vi "sv_UFF58 Set Ordinate Unit and Label.vi"(0 "engineering units":T1=1 items=["custom..."=0, "V"=1, "A"=21, "C"=30, "pC"=31, "s"=32, "-"=29, "Pa"=2, "N"=20, "g"=3, "m/s^2"=4, "m/s"=5, "m"=6, "mm/s"=12, "mm"=13, "micron/s"=14, "micron"=15, "in/s^2"=7, "in/s"=8, "in"=9, "mil/s"=10, "mil"=11, "rad/s^2"=16, "rad/s"=17, "rad"=18, "deg/s^2"=26, "deg/s"=27, "deg"=28, "RPM"=22, "cycle/s^2"=23, "Hz"=24, "cycle"=25, "strain"=19], 7 "unit label":string) -> (4 "ordinate data characteristics (record 9 or 10)":T2={"specific data type"=0, "length units exponent"=0, "force units exponent"=0, "temperature units exponent"=0, "axis label"="NONE", "axis units label"="NONE"} {"specific data type" items=["unknown"=0, "general"=1, "stress"=2, "strain"=3, "temperature"=5, "heat flux"=6, "displacement"=8, "reaction force"=9, "velocity"=11, "acceleration"=12, "excitation force"=13, "pressure"=15, "mass"=16, "time"=17, "frequency"=18, "rpm"=19, "order"=20, "sound pressure"=21, "sound intensity"=22, "sound power"=23]})   [LabVIEW 2017, in "SoundVib_UFF58.lvlib"]
doc: "This VI uses the <B>engineering units</B> from the spectrum info to set the specific data type in the <B>ordinate data characteristics (record 9 or 10)</B>. It also sets the axis label and unit label in the <B>ordinate data characteristics (record 9 or 10)</B>."
uses:
  <vilib>/addons/Sound and Vibration/svt_UFF58/SoundVib_UFF58.lvlib
  <vilib>/addons/Sound and Vibration/svt_UFF58/subVIs/sv_UFF58 Axis Characteristics.ctl
  <vilib>/addons/Sound and Vibration/svt_UFF58/subVIs/sv_UFF58 Specific Datatype.ctl
  <vilib>/addons/_NISVFA/_Shared subVIs/Controls/svc_Engineering Units Text Ring.ctl
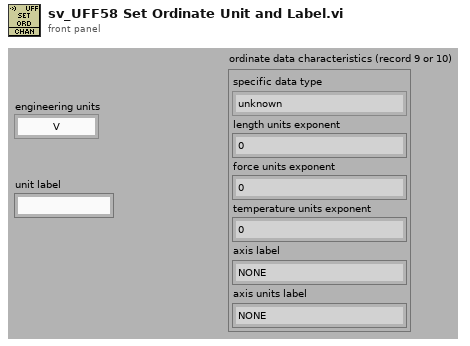
[diagram p1: front panel]
types:
  T1 = typedef "svc_Engineering Units Text Ring.ctl" = u16
  T2 = typedef "SoundVib_UFF58.lvlib/sv_UFF58 Axis Characteristics.ctl" = cluster{"specific data type":T3, "length units exponent":i32, "force units exponent":i32, "temperature units exponent":i32, "axis label":string, "axis units label":string}
  T3 = typedef "SoundVib_UFF58.lvlib/sv_UFF58 Specific Datatype.ctl" = u16
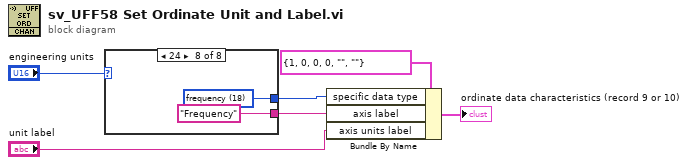
[diagram p0: block diagram]
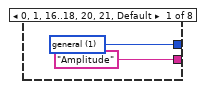
[diagram p2: hidden frame]
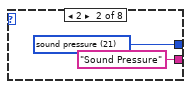
[diagram p3: hidden frame]
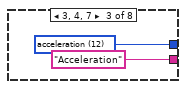
[diagram p4: hidden frame]
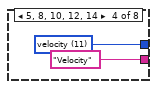
[diagram p5: hidden frame]
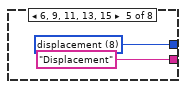
[diagram p6: hidden frame]
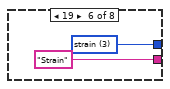
[diagram p7: hidden frame]
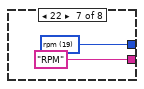
[diagram p8: hidden frame]
diagram:
  n1 = case shown="24" "engineering units" {
    tunnel: [w8 w10 w12 w14 w16 w18 w20 w22] -> w2
    tunnel: ["Amplitude" "Sound Pressure" "Acceleration" "Velocity" "Displacement" "Strain" "RPM" "Frequency"] -> w1
    frame 0, 1, 16..18, 20, 21, Default {
      w8 = T3 1 items=["unknown"=0, "general"=1, "stress"=2, "strain"=3, "temperature"=5, "heat flux"=6, "displacement"=8, "reaction force"=9, "velocity"=11, "acceleration"=12, "excitation force"=13, "pressure"=15, "mass"=16, "time"=17, "frequency"=18, "rpm"=19, "order"=20, "sound pressure"=21, "sound intensity"=22, "sound power"=23] ("specific data type ref")
    }
    frame 2 {
      w10 = T3 21 items=["unknown"=0, "general"=1, "stress"=2, "strain"=3, "temperature"=5, "heat flux"=6, "displacement"=8, "reaction force"=9, "velocity"=11, "acceleration"=12, "excitation force"=13, "pressure"=15, "mass"=16, "time"=17, "frequency"=18, "rpm"=19, "order"=20, "sound pressure"=21, "sound intensity"=22, "sound power"=23] ("specific data type")
    }
    frame 3, 4, 7 {
      w12 = T3 12 items=["unknown"=0, "general"=1, "stress"=2, "strain"=3, "temperature"=5, "heat flux"=6, "displacement"=8, "reaction force"=9, "velocity"=11, "acceleration"=12, "excitation force"=13, "pressure"=15, "mass"=16, "time"=17, "frequency"=18, "rpm"=19, "order"=20, "sound pressure"=21, "sound intensity"=22, "sound power"=23] ("specific data type")
    }
    frame 5, 8, 10, 12, 14 {
      w14 = T3 11 items=["unknown"=0, "general"=1, "stress"=2, "strain"=3, "temperature"=5, "heat flux"=6, "displacement"=8, "reaction force"=9, "velocity"=11, "acceleration"=12, "excitation force"=13, "pressure"=15, "mass"=16, "time"=17, "frequency"=18, "rpm"=19, "order"=20, "sound pressure"=21, "sound intensity"=22, "sound power"=23] ("specific data type")
    }
    frame 6, 9, 11, 13, 15 {
      w16 = T3 8 items=["unknown"=0, "general"=1, "stress"=2, "strain"=3, "temperature"=5, "heat flux"=6, "displacement"=8, "reaction force"=9, "velocity"=11, "acceleration"=12, "excitation force"=13, "pressure"=15, "mass"=16, "time"=17, "frequency"=18, "rpm"=19, "order"=20, "sound pressure"=21, "sound intensity"=22, "sound power"=23] ("specific data type")
    }
    frame 19 {
      w18 = T3 3 items=["unknown"=0, "general"=1, "stress"=2, "strain"=3, "temperature"=5, "heat flux"=6, "displacement"=8, "reaction force"=9, "velocity"=11, "acceleration"=12, "excitation force"=13, "pressure"=15, "mass"=16, "time"=17, "frequency"=18, "rpm"=19, "order"=20, "sound pressure"=21, "sound intensity"=22, "sound power"=23] ("specific data type")
    }
    frame 22 {
      w20 = T3 19 items=["unknown"=0, "general"=1, "stress"=2, "strain"=3, "temperature"=5, "heat flux"=6, "displacement"=8, "reaction force"=9, "velocity"=11, "acceleration"=12, "excitation force"=13, "pressure"=15, "mass"=16, "time"=17, "frequency"=18, "rpm"=19, "order"=20, "sound pressure"=21, "sound intensity"=22, "sound power"=23] ("specific data type")
    }
    frame 24 {
      w22 = T3 18 items=["unknown"=0, "general"=1, "stress"=2, "strain"=3, "temperature"=5, "heat flux"=6, "displacement"=8, "reaction force"=9, "velocity"=11, "acceleration"=12, "excitation force"=13, "pressure"=15, "mass"=16, "time"=17, "frequency"=18, "rpm"=19, "order"=20, "sound pressure"=21, "sound intensity"=22, "sound power"=23] ("specific data type")
    }
  }
  n2 = Bundle By Name(cluster=T2 {"specific data type"=1, "length units exponent"=0, "force units exponent"=0, "temperature units exponent"=0, "axis label"="", "axis units label"=""} ("abscissa data characteristics"), "specific data type"=w2, "axis label"=w1, "axis units label"="unit label") -> (→"ordinate data characteristics (record 9 or 10)":T2)
